vi "Pre Launch Init.vi"(11 "UI Base in":refnum<class "UI Base.lvclass">) -> (0 "error out":errorcluster, 3 "UI Base out":refnum<class "UI Base.lvclass">)   [LabVIEW 2023, in "UI Base.lvlib" / "UI Base.lvclass"]
doc: "(<B>Filename</B>: Actor Framework.lvlib:Actor.lvclass:Pre Launch Init.vi)\n\nDefines behavior that occurs after the Launch Nested Actor method is invoked but before the actor's Actor Core method begins running.\n\nBy default, this method does nothing. A descendant class may override it to define behavior."
uses:
  UI Base.lvclass
  UI Base.lvclass/UI Base.ctl
  <vilib>/ActorFramework/Actor/Actor.lvclass
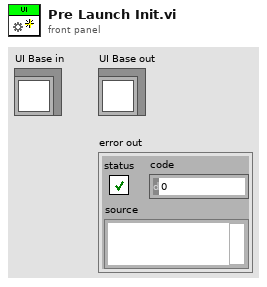
[diagram p1: front panel]
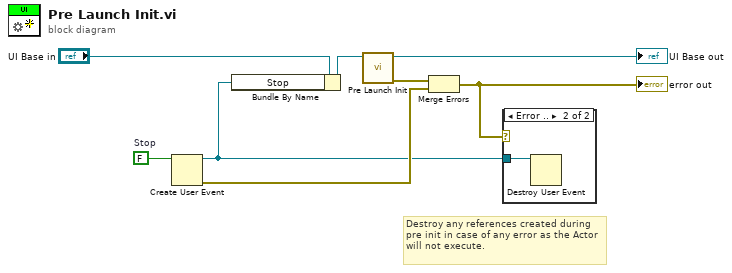
[diagram p0: block diagram]
diagram:
  w7 = FALSE  # Stop
  # "Destroy any references created during pre init in case of any error as the Actor will not execute."
  n1 = Create User Event(user event datatype=w7) -> (user event=w4:refnum<user-event>, error out=w5:errorcluster)  [unwired: 1 in]
  n2 = Bundle By Name(cluster="UI Base in", "Stop"=w4) -> (w6:refnum<class "UI Base.lvclass">)
  n3 = call-parent "Pre Launch Init.vi"("Actor in"=w6) -> ("error out"=w8:errorcluster, "Actor out"=→"UI Base out":refnum<class "UI Base.lvclass">)  [unwired: 9 in]
  n4 = Merge Errors(w8, w5) -> (w1:errorcluster)
  "error out" <- w1
  n5 = case shown="Error .." w1 {
    tunnel: w4 -> [_ w9]
    frame No Error {
    }
    frame Error {
      n6 = Destroy User Event(user event=w9) -> ()  [unwired: 1 in, 1 out]
    }
  }
